vi "Sequencer UI - Start Here.vi"() -> ()   [LabVIEW 2019]
uses:
  typedefs/step.data--Cluster.ctl
  typedefs/step.IO.data--Cluster.ctl
  typedefs/IOType--Enum.ctl
panel:
  in  "Sequence MCL Ref":i32(listbox) caption="Sequence"
  in  "Abort Sequence":bool
  in  "Run Sequence":bool
  in  "Load Sequence":bool
  in  "Exit":bool
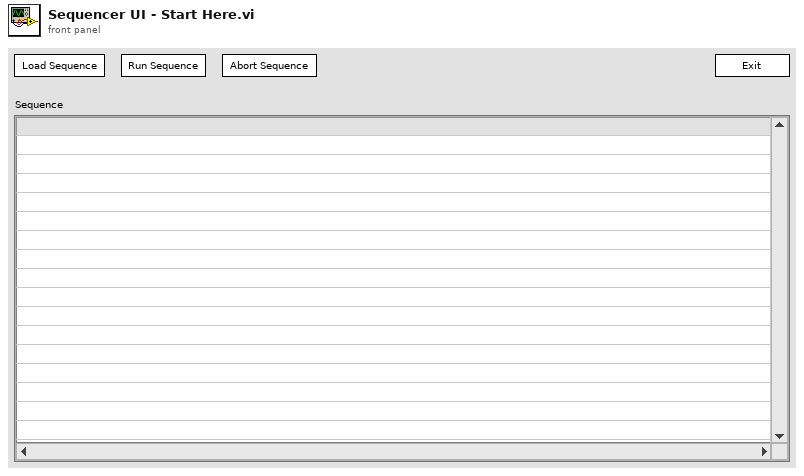
[diagram p1: front panel]
types:
  T1 = enum32{"invalid app kind", "Development System", "Run Time System", "Student Edition", "Embedded LabVIEW", "Evaluation", "Custom"}
  T2 = enum32{"Invalid", "Standard", "Closed", "Hidden", "Minimized", "Maximized"}
  T3 = typedef "step.data--Cluster.ctl" = cluster{"Step ID":string, "Dwell Time(s)":dbl, "Recipe Step":T4[]}
  T4 = typedef "step.IO.data--Cluster.ctl" = cluster{"IO Name":string, "IO Type":T5, "IO Value":variant}
  T5 = typedef "IOType--Enum.ctl" = enum16{"<Undefined>", "DO", "DI", "AO", "AI"}
  T6 = cluster{"Core":cluster{"Current VI Reference":refnum<vi>, "Close Panel on Exit?":bool}, "Your Boolean data":bool, "Your string data":string, "Sequence Data [ ]":T3[], "Sequence MCL Ref":refnum<vi>}
  T7 = cluster{"Current VI Reference":refnum<vi>, "Close Panel on Exit?":bool}
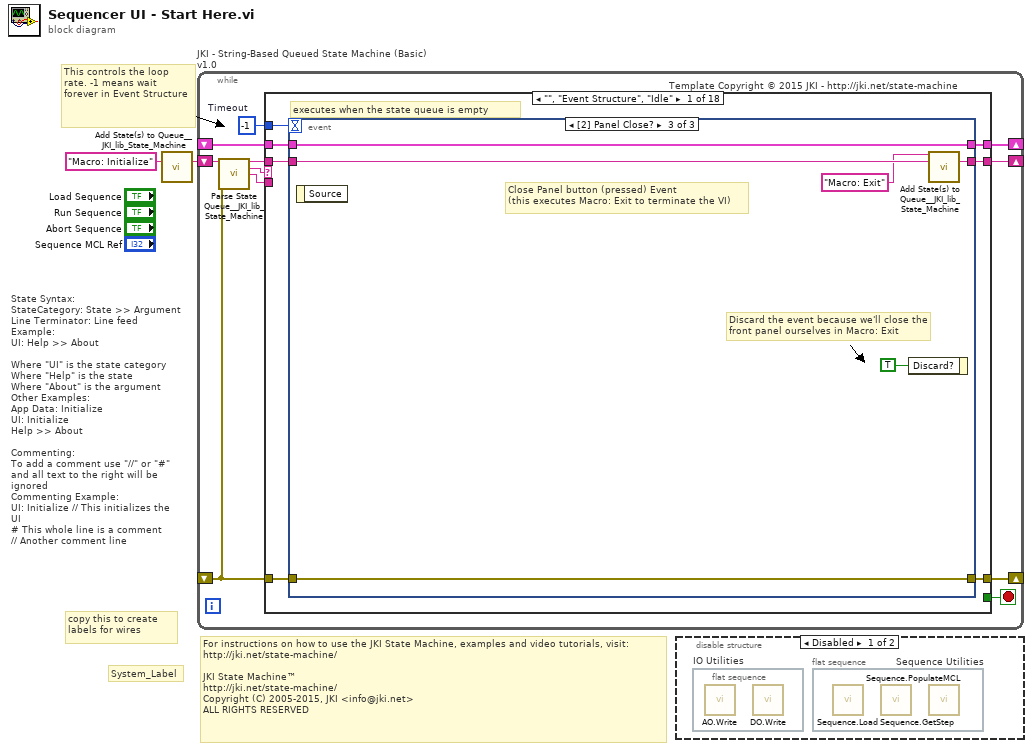
[diagram p0: block diagram]
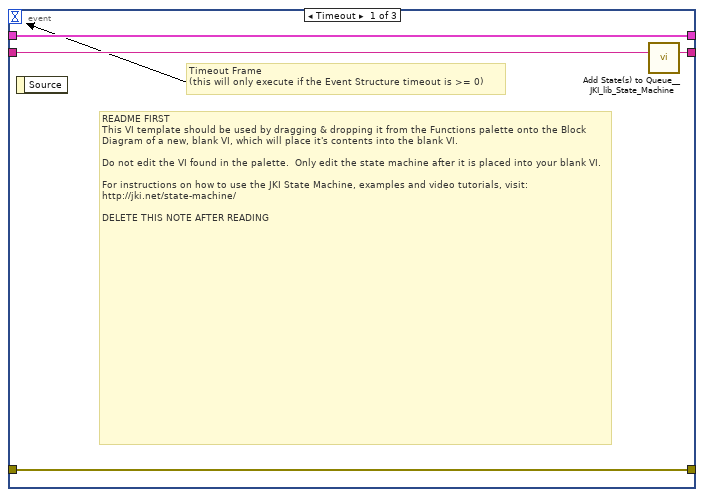
[diagram p3: hidden frame]
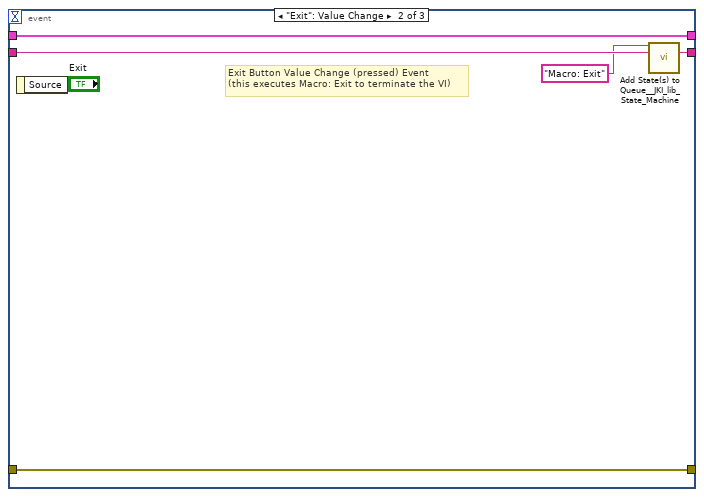
[diagram p4: hidden frame]
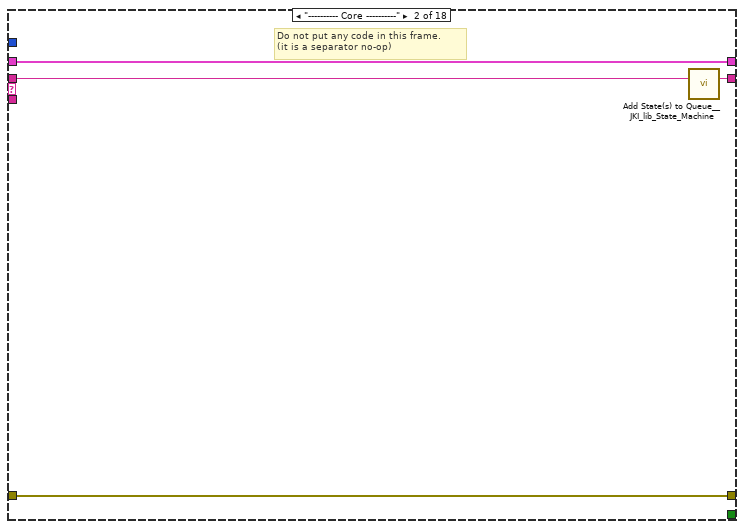
[diagram p5: hidden frame]
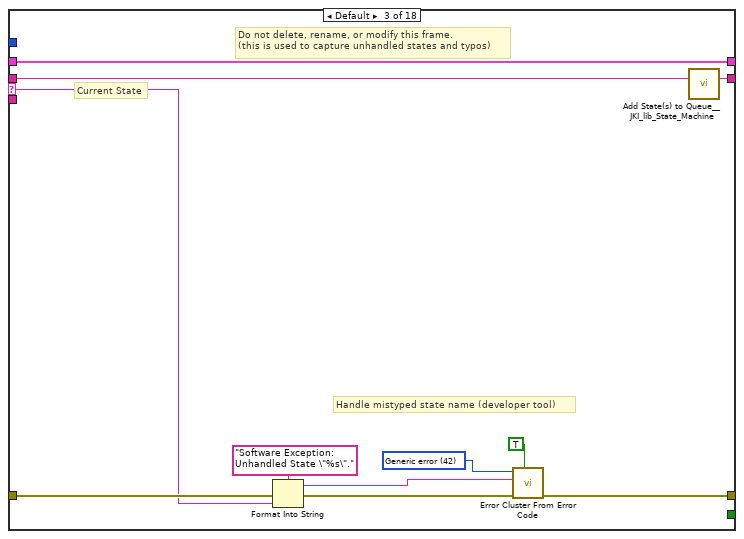
[diagram p6: hidden frame]
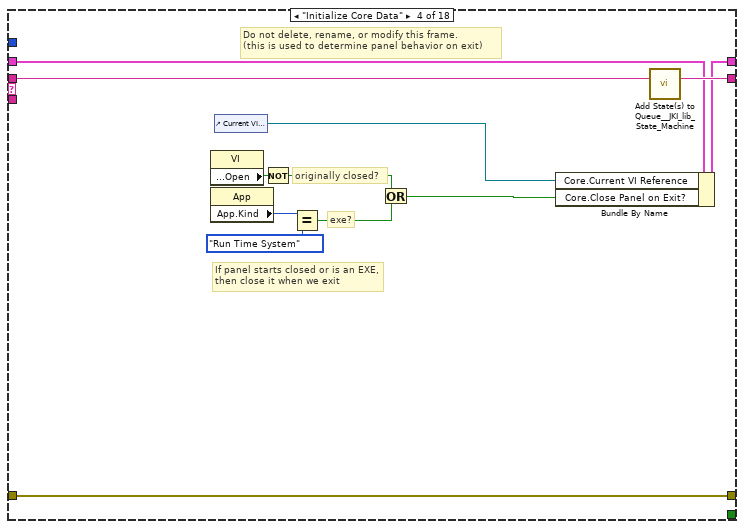
[diagram p7: hidden frame]
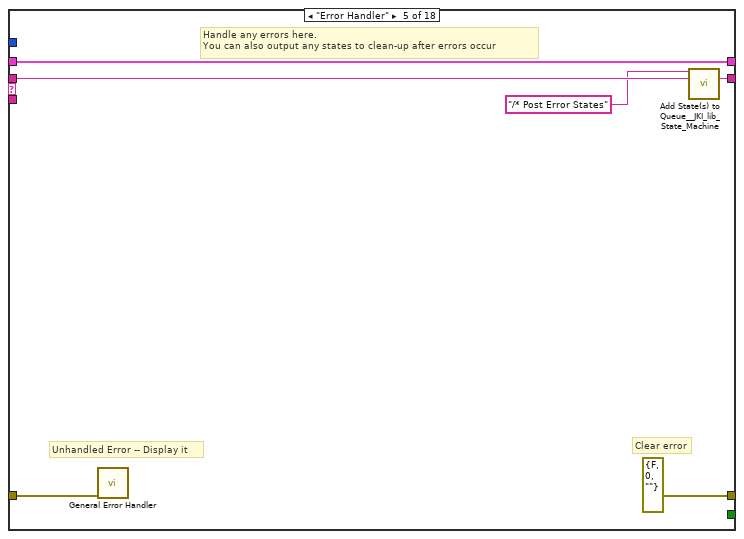
[diagram p8: hidden frame]
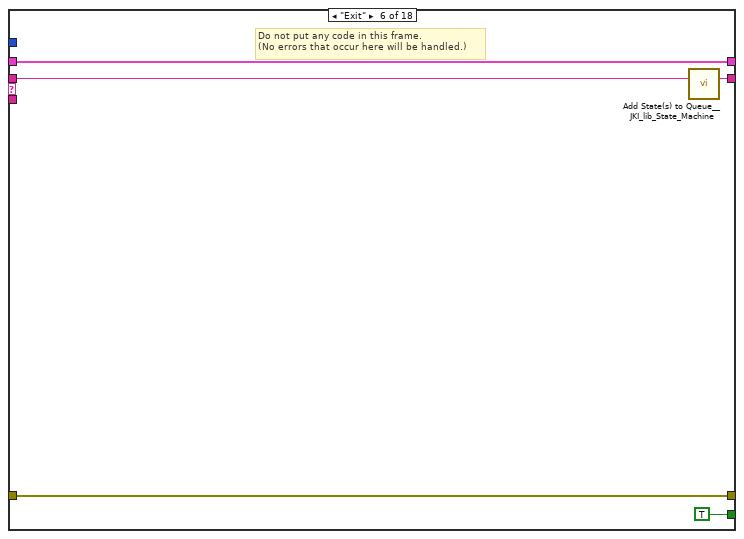
[diagram p9: hidden frame]
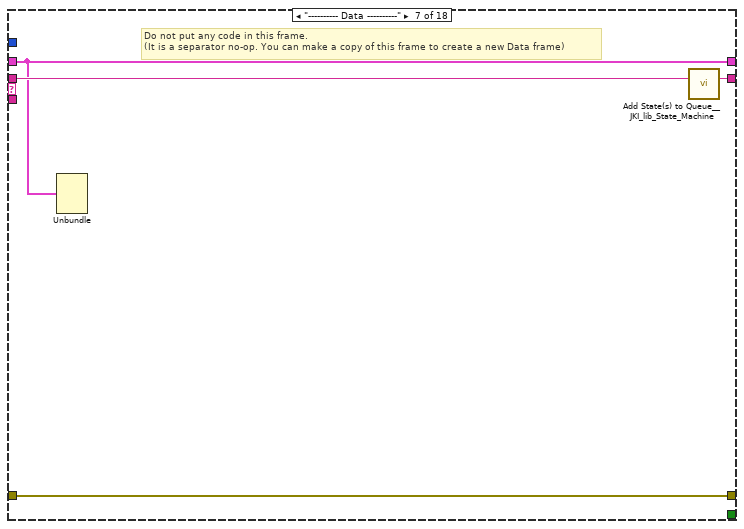
[diagram p10: hidden frame]
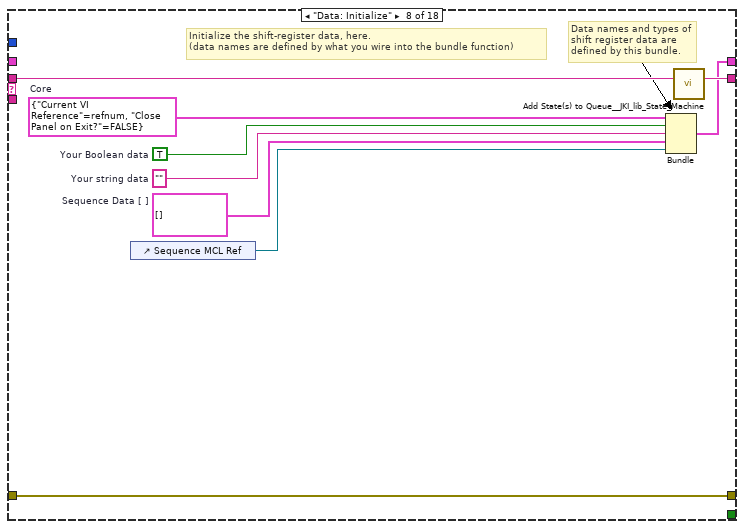
[diagram p11: hidden frame]
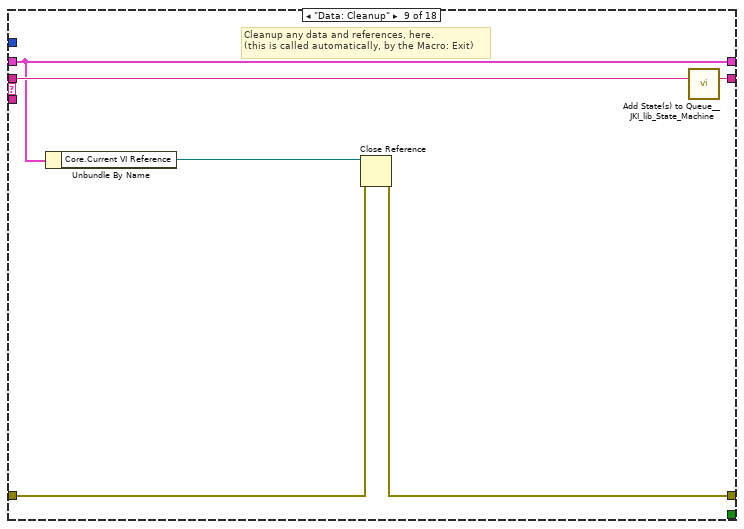
[diagram p12: hidden frame]
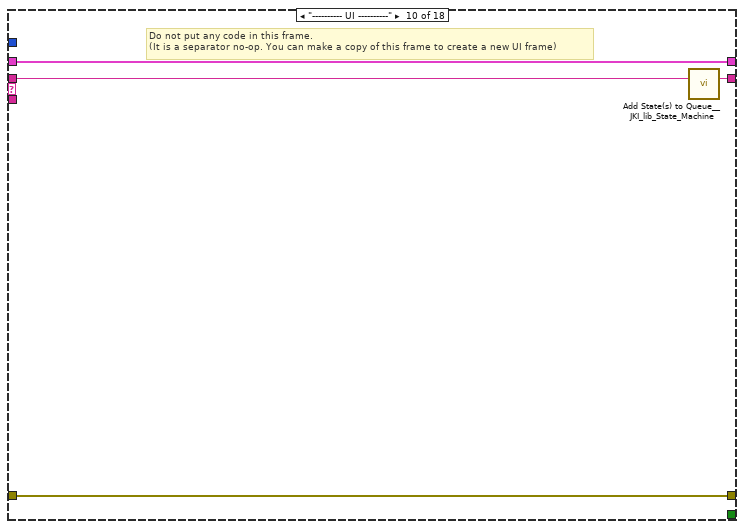
[diagram p13: hidden frame]
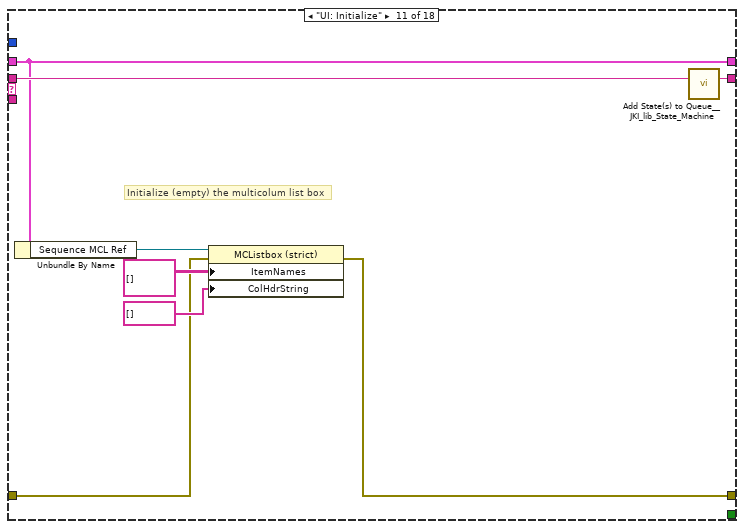
[diagram p14: hidden frame]
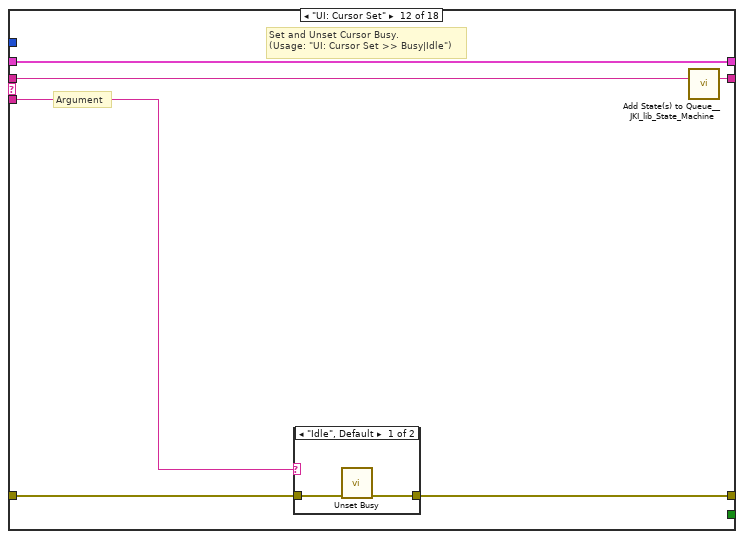
[diagram p15: hidden frame]
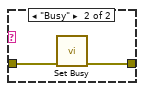
[diagram p16: hidden frame]
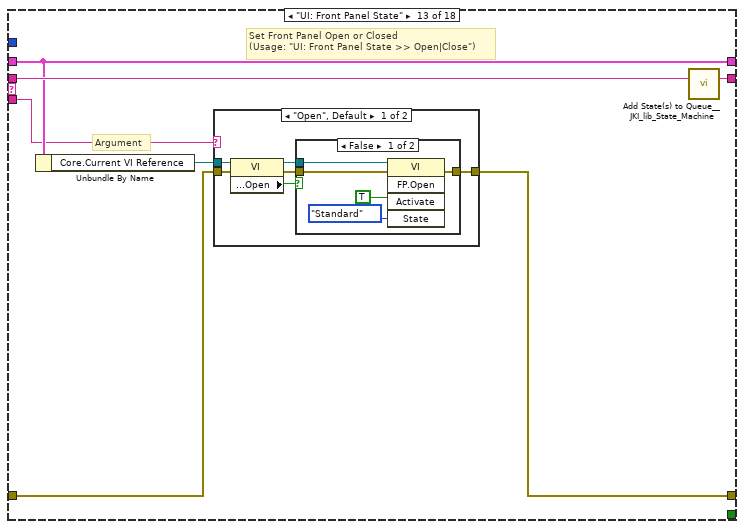
[diagram p17: hidden frame]
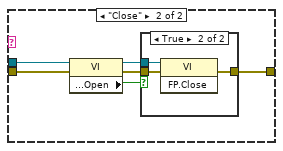
[diagram p19: hidden frame]
diagram:
  # "For instructions on how to use the JKI State Machine, examples and video tutorials, visit:\nhttp://jki.net/state-machine/\n\nJKI State Machine™\nhttp://jki.net/state-machine/\nCopyright (C) 2005-2015, JKI <info@jki.net>\nALL RIGHTS RESERVED"
  # "State Syntax:\nStateCategory: State >> Argument\nLine Terminator: Line feed\nExample:\nUI: Help >> About\n\nWhere \"UI\" is the state category\nWhere \"Help\" is the state\nWhere \"About\" is the argument\nOther Examples:\nApp Data: Initialize\nUI: Initialize\nHelp >> About\n\nCommenting:\nTo add a comment use \"//\" or \"#\" and all text to the right will be ignored\nCommenting Example:\nUI: Initialize // This initializes the UI\n# This whole line is a comment\n// Another comment line"
  # "copy this to create labels for wires"
  # "This controls the loop rate. -1 means wait forever in Event Structure"
  # "System_Label"
  n1 = call <vilib>:"Add State(s) to Queue__JKI_lib_State_Machine.vi"("State(s) in (\"\")"="Macro: Initialize") -> ("States Out"=w2:string)  [unwired: 14 in]
  n2 = while "JKI - String-Based Queued State Machine (Basic) v1.0" {
    shift-right: [w6] -> _
    shift-left: _ -> [w5]
    shift-right: [w9] -> _
    shift-left: _ -> [w3]
    shift-right: [w8] -> _
    shift-left: w2 -> [w10]
    stop <- w7 stop-if-true
    w4 = -1  # Timeout
    # "Template Copyright © 2015 JKI - http://jki.net/state-machine"
    n3 = call <vilib>:"Parse State Queue__JKI_lib_State_Machine.vi"("State Queue"=w10, "Error In (no error)"=w3) -> ("Remaining States"=w12:string, "Current State"=w13:string, "Arguments"=w11:string)  [unwired: 11 in]
    n4 = case shown="\"\", \"Event Structure\", \"Idle\"" w13 {
      selector: w13 -> [_ _ w40 _ _ _ _ _ _ _ _ _ _ _ _ _ _ _]
      tunnel: w12 -> [w20 w39 w44 w62 w68 w73 w77 w86 w92 w96 w104 w110 w121 w147 w152 w162 w166 w170]
      tunnel: w11 -> [_ _ _ _ _ _ _ _ _ _ _ w105 w115 _ _ _ _ _]
      tunnel: w5 -> [w18 w36 w42 w53 w65 w71 w74 _ w87 w93 w102 w108 w117 w144 w149 w159 w163 w167]
      tunnel: [w17 w37 w46 w59 errorcluster {"status"=FALSE, "code"=0, "source"=""} ("error out") w70 w75 w83 w88 w94 w97 w106 w118 w145 w150 w160 w164 w168] -> w9
      tunnel: w3 -> [w16 w37 w45 w59 w64 w70 w75 w83 w89 w94 w98 w107 w119 w145 w150 w160 w164 w168]
      tunnel: [w19 w38 w43 w61 w67 w72 w76 w85 w91 w95 w103 w109 w120 w146 w151 w161 w165 w169] -> w8
      tunnel: [_ _ _ _ _ TRUE _ _ _ _ _ _ _ _ _ _ _ _] -> w7
      tunnel: [w15 w36 w42 w60 w65 w71 w74 w84 w87 w93 w102 w108 w117 w144 w149 w159 w163 w167] -> w6
      tunnel: w4 -> [w14 _ _ _ _ _ _ _ _ _ _ _ _ _ _ _ _ _]
      frame "", "Event Structure", "Idle" {
        # "executes when the state queue is empty"
        n5 = event shown="[2] Panel Close?" {
          selector: _ -> [_ _ _]
          dyn-events: _ -> [_ _ _]
          timeout: w14 -> [_ _ _]
          tunnel: w20 -> [w24 w29 w35]
          tunnel: [w23 w28 w34] -> w19
          tunnel: w18 -> [w21 w26 w32]
          tunnel: [w22 w27 w33] -> w17
          tunnel: w16 -> [w22 w27 w33]
          tunnel: [w21 w26 w32] -> w15
          event Timeout {
            # "README FIRST\nThis VI template should be used by dragging & dropping it from the Functions palette onto the Block Diagram of a new, blank VI, which will place it's contents into the blank VI.\n\nDo not edit the VI found in the palette.  Only edit the state machine after it is placed into your blank VI.\n\nFor instructions on how to use the JKI State Machine, examples and video tutorials, visit:\nhttp://jki.net/state-machine/\n\nDELETE THIS NOTE AFTER READING"
            # "Timeout Frame\n(this will only execute if the Event Structure timeout is >= 0)"
            n6 = event-data() -> ()  [unwired: 1 in, 1 out]
            n7 = call <vilib>:"Add State(s) to Queue__JKI_lib_State_Machine.vi"("State(s) in (\"\")"=w24) -> ("States Out"=w23:string)  [unwired: 14 in]
          }
          event "Exit": Value Change {
            # "Exit Button Value Change (pressed) Event\n(this executes Macro: Exit to terminate the VI)"
            n8 = event-data() -> ()  [unwired: 1 in, 1 out]
            n9 = call <vilib>:"Add State(s) to Queue__JKI_lib_State_Machine.vi"("State(s) in Front (\"\")"="Macro: Exit", "State(s) in (\"\")"=w29) -> ("States Out"=w28:string)  [unwired: 13 in]
          }
          event Panel Close? {
            # "Discard the event because we'll close the front panel ourselves in Macro: Exit"
            # "Close Panel button (pressed) Event\n(this executes Macro: Exit to terminate the VI)"
            n10 = event-data() -> ()  [unwired: 1 in, 1 out]
            n11 = event-data("Discard?"=TRUE) -> ()  [unwired: 1 in, 1 out]
            n12 = call <vilib>:"Add State(s) to Queue__JKI_lib_State_Machine.vi"("State(s) in Front (\"\")"="Macro: Exit", "State(s) in (\"\")"=w35) -> ("States Out"=w34:string)  [unwired: 13 in]
          }
        }
      }
      frame "---------- Core ----------" {
        # "Do not put any code in this frame.\n(it is a separator no-op)"
        n13 = call <vilib>:"Add State(s) to Queue__JKI_lib_State_Machine.vi"("State(s) in (\"\")"=w39) -> ("States Out"=w38:string)  [unwired: 14 in]
      }
      frame Default {
        w49 = 42 items=["No error", "Argument error", "Memory is full", "Out of zone", "End of file", "File already open", "Generic file I/O error", "File not found", "File permission error", "Disk is full", "Duplicate path", "Too many files open", "System feature not enabled", "Resource file not found", "Cannot add resource", "Resource not found", "Image not found", "Image memory error", "Pen does not exist", "Config type invalid", "Config token not found", "Config parse error", "Config memory error", "Bad external code format", "Bad external code offset", "External code not present", "Null window", "Destroy window error", "Null menu", "Print aborted", "Bad print record", "Print driver error", "Windows error during printing", "Memory error during printing", "Print dialog error", "Generic print error", "Invalid device refnum", "Device not found", "Device parameter error", "Device unit error", "Cannot open device", "Device call aborted", "Generic error", "Cancelled by user", "Object ID too low", "Object ID too high", "Object not in heap", "Unknown heap", "Unknown object (invalid DefProc)", "Unknown object (DefProc not in table)", "Message out of range", "Invalid (null) method", "Unknown message", "Manager call not supported", "Bad address", "Network operation in progress", "Network operation timed out", "Connection is busy", "Network attribute not supported", "Network error", "Address in use", "System out of memory", "Connection aborted", "Connection refused", "Not connected", "Already connected", "Connection closed", "Initialization error (interapplication manager)", "Bad occurrence", "Wait on unbound occurrence handler", "Occurrence queue overflow", "Datalog type conflict", "Unused", "Unrecognized type (interapplication manager)", "Memory corrupt", "Failed to make temporary DLL", "Old CIN version", "Drag socket not found", "Failed to load drop-object", "Failed to register OLE object", "Failed to release OLE object", "Format specifier type mismatch", "Unknown format specifier", "Too few format specifiers", "Too many format specifiers", "Scan failed", "Newer CIN version", "Error converting to variant", "Runtime menu error", "Password tampered", "Variant attribute not found", "Incompatible variant data type", "Event data is not available", "Event Store is not present", "Occurrence is not found", "Event Queue is not created", "Event info is not available", "Refnum passed is NULL", "Error retrieving Class GUID", "Error retrieving CoClass GUID", "Error retrieving TypeLib GUID.", "Bad built application magic bytes.", "Specific driver is different from the specific driver associated with the Logical Name.", "There is no session opened to the class driver.", "Max Error", "MAX - Error with config objects", "MAX - Error loading configuration", "MAX - Group not supported"]
        # "Current State"
        # "Do not delete, rename, or modify this frame.\n(this is used to capture unhandled states and typos)"
        # "Handle mistyped state name (developer tool)"
        n14 = Format Into String(format string="Software Exception: Unhandled State \"%s\"." ("message"), error in=w45, w40) -> (resulting string=w48:string, error out=w47:errorcluster)  [unwired: 1 in]
        n15 = call <vilib>:"Error Cluster From Error Code.vi"("show call chain? (False)"=TRUE, "error in (no error)"=w47, "error message (\"\")"=w48, "error code (0)"=w49) -> ("error out"=w46:errorcluster)  [unwired: 5 in]
        n16 = call <vilib>:"Add State(s) to Queue__JKI_lib_State_Machine.vi"("State(s) in (\"\")"=w44) -> ("States Out"=w43:string)  [unwired: 14 in]
      }
      frame "Initialize Core Data" {
        # "Do not delete, rename, or modify this frame.\n(this is used to determine panel behavior on exit)"
        # "originally closed?"
        # "exe?"
        # "If panel starts closed or is an EXE, then close it when we exit"
        n17 = property class="VI"() -> ("Front Panel.Open"=w58:bool)  [unwired: 2 in, 2 out]
        n18 = property class="App"() -> ("App.Kind"=w57:T1)  [unwired: 2 in, 2 out]
        n19 = control-ref of="Current VI Reference"() -> (w51:refnum<vi>)
        n20 = Not(x=w58) -> (.not. x?=w55:bool)
        n21 = Equal?(x=w57, y=T1."Run Time System" ("Application:Kind")) -> (x = y?=w54:bool)
        n22 = Or(x=w55, y=w54) -> (x .or. y?=w52:bool)
        n23 = Bundle By Name(cluster=w53, "Core.Current VI Reference"=w51, "Core.Close Panel on Exit?"=w52) -> (w60:T6)
        n24 = call <vilib>:"Add State(s) to Queue__JKI_lib_State_Machine.vi"("State(s) in (\"\")"=w62) -> ("States Out"=w61:string)  [unwired: 14 in]
      }
      frame "Error Handler" {
        # "Unhandled Error -- Display it"
        # "Handle any errors here.\nYou can also output any states to clean-up after errors occur"
        # "Clear error"
        n25 = call <vilib>:"General Error Handler.vi"("error in (no error)"=w64) -> ()  [unwired: 10 in, 5 out]
        n26 = call <vilib>:"Add State(s) to Queue__JKI_lib_State_Machine.vi"("State(s) in Front (\"\")"="/* Post Error States", "State(s) in (\"\")"=w68) -> ("States Out"=w67:string)  [unwired: 13 in]
      }
      frame "Exit" {
        # "Do not put any code in this frame.\n(No errors that occur here will be handled.)"
        n27 = call <vilib>:"Add State(s) to Queue__JKI_lib_State_Machine.vi"("State(s) in (\"\")"=w73) -> ("States Out"=w72:string)  [unwired: 14 in]
      }
      frame "---------- Data ----------" {
        # "Do not put any code in this frame.\n(It is a separator no-op. You can make a copy of this frame to create a new Data frame)"
        n28 = Unbundle(w74) -> ()  [unwired: 5 out]
        n29 = call <vilib>:"Add State(s) to Queue__JKI_lib_State_Machine.vi"("State(s) in (\"\")"=w77) -> ("States Out"=w76:string)  [unwired: 14 in]
      }
      frame "Data: Initialize" {
        w79 = T3[] []  # Sequence Data [ ]
        w80 = T7 {"Current VI Reference"=refnum, "Close Panel on Exit?"=FALSE}  # Core
        w82 = TRUE  # Your Boolean data
        w81 = ""  # Your string data
        # "Data names and types of shift register data are defined by this bundle."
        # "Initialize the shift-register data, here.\n(data names are defined by what you wire into the bundle function)"
        n30 = control-ref of="Sequence MCL Ref"() -> (w78:refnum<vi>)
        n31 = Bundle("Core"=w80, "Your Boolean data"=w82, "Your string data"=w81, "Sequence Data [ ]"=w79, "Sequence MCL Ref"=w78) -> (w84:T6)  [unwired: 1 in]
        n32 = call <vilib>:"Add State(s) to Queue__JKI_lib_State_Machine.vi"("State(s) in (\"\")"=w86) -> ("States Out"=w85:string)  [unwired: 14 in]
      }
      frame "Data: Cleanup" {
        # "Cleanup any data and references, here.\n(this is called automatically, by the Macro: Exit)"
        n33 = Unbundle By Name(w87) -> ("Core.Current VI Reference"=w90:refnum<vi>)
        n34 = Close Reference(reference=w90, error in (no error)=w89) -> (error out=w88:errorcluster)
        n35 = call <vilib>:"Add State(s) to Queue__JKI_lib_State_Machine.vi"("State(s) in (\"\")"=w92) -> ("States Out"=w91:string)  [unwired: 14 in]
      }
      frame "---------- UI ----------" {
        # "Do not put any code in this frame.\n(It is a separator no-op. You can make a copy of this frame to create a new UI frame)"
        n36 = call <vilib>:"Add State(s) to Queue__JKI_lib_State_Machine.vi"("State(s) in (\"\")"=w96) -> ("States Out"=w95:string)  [unwired: 14 in]
      }
      frame "UI: Initialize" {
        # "Initialize (empty) the multicolum list box"
        n37 = Unbundle By Name(w102) -> ("Sequence MCL Ref"=w101:refnum<vi>)
        n38 = property class="MCListbox (strict)"(reference=w101, error in=w98, "ItemNames"=string[][] [] ("Item Names"), "ColHdrString"=string[] [] ("Column Header Strings[]")) -> (error out=w97:errorcluster)  [unwired: 1 out]
        n39 = call <vilib>:"Add State(s) to Queue__JKI_lib_State_Machine.vi"("State(s) in (\"\")"=w104) -> ("States Out"=w103:string)  [unwired: 14 in]
      }
      frame "UI: Cursor Set" {
        # "Argument"
        # "Set and Unset Cursor Busy.\n(Usage: \"UI: Cursor Set >> Busy|Idle\")"
        n40 = case shown="\"Idle\", Default" w105 {
          tunnel: w107 -> [w112 w114]
          tunnel: [w111 w113] -> w106
          frame "Idle", Default {
            n41 = call <vilib>:"Unset Busy.vi"("error in (no error)"=w112) -> ("error out"=w111:errorcluster)  [unwired: 10 in]
          }
          frame "Busy" {
            n42 = call <vilib>:"Set Busy.vi"("error in (no error)"=w114) -> ("error out"=w113:errorcluster)  [unwired: 9 in, 1 out]
          }
        }
        n43 = call <vilib>:"Add State(s) to Queue__JKI_lib_State_Machine.vi"("State(s) in (\"\")"=w110) -> ("States Out"=w109:string)  [unwired: 14 in]
      }
      frame "UI: Front Panel State" {
        # "Argument"
        # "Set Front Panel Open or Closed\n(Usage: \"UI: Front Panel State >> Open|Close\")"
        n44 = Unbundle By Name(w117) -> ("Core.Current VI Reference"=w116:refnum<vi>)
        n45 = case shown="\"Open\", Default" w115 {
          tunnel: w119 -> [w125 w138]
          tunnel: [w127 w139] -> w118
          tunnel: w116 -> [w126 w136]
          frame "Open", Default {
            n46 = property class="VI"(reference=w126, error in=w125) -> (reference out=w123:refnum<vi>, error out=w124:errorcluster, "Front Panel.Open"=w122:bool)
            n47 = case shown="False" w122 {
              tunnel: [w130 w133] -> w127
              tunnel: w124 -> [w129 w133]
              tunnel: w123 -> [w128 _]
              frame False {
                n48 = invoke class="VI" method="FP.Open"(reference=w128, error in=w129, "Activate"=TRUE, "State"=T2."Standard") -> (error out=w130:errorcluster)  [unwired: 1 in, 4 out]
              }
              frame True {
              }
            }
          }
          frame "Close" {
            n49 = property class="VI"(reference=w136, error in=w138) -> (reference out=w135:refnum<vi>, error out=w137:errorcluster, "Front Panel.Open"=w134:bool)
            n50 = case shown="True" w134 {
              tunnel: [w140 w143] -> w139
              tunnel: w137 -> [w140 w142]
              tunnel: w135 -> [_ w141]
              frame False {
              }
              frame True {
                n51 = invoke class="VI" method="FP.Close"(reference=w141, error in=w142) -> (error out=w143:errorcluster)  [unwired: 1 in, 2 out]
              }
            }
          }
        }
        n52 = call <vilib>:"Add State(s) to Queue__JKI_lib_State_Machine.vi"("State(s) in (\"\")"=w121) -> ("States Out"=w120:string)  [unwired: 14 in]
      }
      frame "---------- Macro ----------" {
        # "Do not put any code in this frame.\n(It is a separator no-op. You can make a copy of this frame to create a new Macro frame)"
        n53 = call <vilib>:"Add State(s) to Queue__JKI_lib_State_Machine.vi"("State(s) in (\"\")"=w147) -> ("States Out"=w146:string)  [unwired: 14 in]
      }
      frame "Macro: Initialize" {
        w148 = "Data: Initialize\nInitialize Core Data\nUI: Initialize\nUI: Front Panel State >> Open"  # Data: Initialize Initialize Core Data UI: Initialize UI: Front Panel State >> Open
        # "Initialization Macro\n(This is called once, when the VI starts)"
        n54 = call <vilib>:"Add State(s) to Queue__JKI_lib_State_Machine.vi"("State(s) in Front (\"\")"=w148, "State(s) in (\"\")"=w152) -> ("States Out"=w151:string)  [unwired: 13 in]
      }
      frame "Macro: Exit" {
        # "Exit Macro\n(This is called once, when the VI exits)"
        n55 = Unbundle By Name(w159) -> ("Core.Close Panel on Exit?"=w158:bool)
        n56 = Select(t="UI: Front Panel State >> Close", s=w158, f="") -> (s? t:f=w155:string)
        n57 = call <vilib>:"Add State(s) to Queue__JKI_lib_State_Machine.vi"("State(s) in (\"\")"=w155, "State(s) at Back (\"\")"="Data: Cleanup\nExit") -> ("States Out"=w153:string)  [unwired: 13 in]
        n58 = call <vilib>:"Add State(s) to Queue__JKI_lib_State_Machine.vi"("State(s) in Front (\"\")"=w153, "State(s) in (\"\")"=w162) -> ("States Out"=w161:string)  [unwired: 13 in]
      }
      frame "---------- IO ----------" {
        # "Template Separator\n(You can make a copy of, or modify, this frame)"
        n59 = call <vilib>:"Add State(s) to Queue__JKI_lib_State_Machine.vi"("State(s) in (\"\")"=w166) -> ("States Out"=w165:string)  [unwired: 14 in]
      }
      frame "---------- Sequence ----------" {
        # "Template Separator\n(You can make a copy of, or modify, this frame)"
        n60 = call <vilib>:"Add State(s) to Queue__JKI_lib_State_Machine.vi"("State(s) in (\"\")"=w170) -> ("States Out"=w169:string)  [unwired: 14 in]
      }
    }
  }
  n61 = disable-structure shown="Disabled" {
    frame Disabled {
      n62 = flat-sequence "IO Utilities" {
        frame #0 {
          n63 = call "AO.Write.vi"() -> ()  [unwired: 11 in, 1 out]
          n64 = call "DO.Write.vi"() -> ()  [unwired: 11 in, 1 out]
        }
      }
      n65 = flat-sequence "Sequence Utilities" {
        frame #0 {
          n66 = call "Sequence.Load.vi"() -> ()  [unwired: 9 in, 3 out]
          n67 = call "Sequence.GetStep.vi"() -> ()  [unwired: 9 in, 3 out]
          n68 = call "Sequence.PopulateMCL.vi"() -> ()  [unwired: 11 in, 1 out]
        }
      }
    }
    frame Enabled {
    }
  }
